vi "公式写入.vi"(7 "公式":cluster{"X^2":dbl, "X":dbl, "b":dbl}, 8 "error in (no error)":errorcluster caption="错误输入（无错误）", 9 "量程":enum16{"低量程", "高量程"}(ring), 10 "测量模式":T1(ring), 11 "测量参数":u16(ring) items=["总磷"=1, "总氮"=2, "氨氮"=3, "COD"=22]) -> (0 "error out":errorcluster caption="错误输出")   [LabVIEW 2016, in "斯坦道总氮.lvlib"]
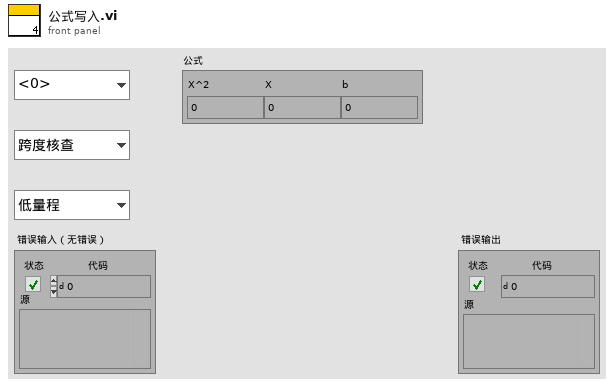
[diagram p1: front panel]
types:
  T1 = enum16{"跨度核查", "水样测量", "零点核查", "标样核查", "加标回收", "平行样测试", "空白校准", "标样校准", "空白测试"}
  T2 = typedef "SingleStepTestV3.lvlib/SingleStepTestV3.lvclass/仪器版本.ctl" = enum16{"V3.1版", "V4版", "V3版", "V4.2版"}
  T3 = cluster{"测量参数":u16, "测量模式":enum16{"跨度核查", "水样测量", "零点核查", "标样核查", "加标回收", "平行样测试", "空白校准", "标样校准", "空白测试"}, "量程":enum16{"低量程", "高量程"}}
  T4 = typedef "斯坦道总氮.lvlib/校准参数.ctl" = cluster{"公式写入时间":timestamp, "id":u8, "fid":u8, "range":u8, "拟合方法":u16, "精度":u16, "公式A":sgl, "公式B":sgl, "公式C":sgl, "R2":sgl, "校准值一":cluster{"标准值":sgl, "吸光值":sgl, "启用":bool, "数据时间":timestamp}, "校准值二":cluster{"标准值":sgl, "吸光值":sgl, "启用":bool, "数据时间":timestamp}, "校准值三":cluster{"标准值":sgl, "吸光值":sgl, "启用":bool, "数据时间":timestamp}, "校准值四":cluster{"标准值":sgl, "吸光值":sgl, "启用":bool, "数据时间":timestamp}, "校准值五":cluster{"标准值":sgl, "吸光值":sgl, "启用":bool, "数据时间":timestamp}}
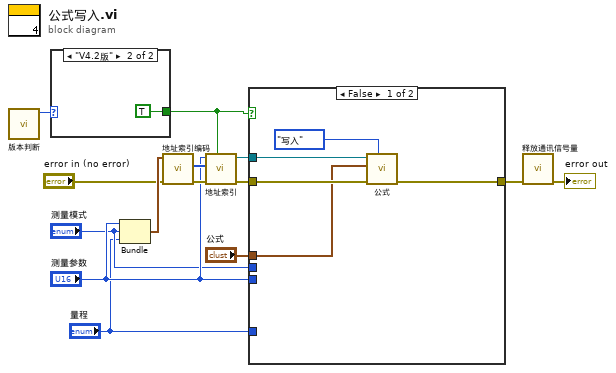
[diagram p0: block diagram]
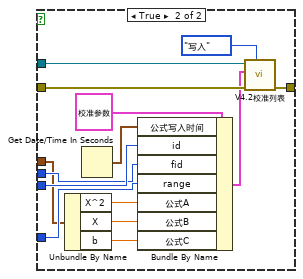
[diagram p2: hidden frame]
diagram:
  n1 = call "版本判断.vi"() -> ("仪器版本"=w9:T2)  [unwired: 11 in]
  n2 = case shown="\"V4.2版\"" w9 {
    tunnel: [_ TRUE] -> w4
    frame "V3.1版", Default {
    }
    frame "V4.2版" {
    }
  }
  n3 = Bundle("测量参数"="测量参数", "测量模式"="测量模式", "量程"="量程") -> (w8:T3)  [unwired: 1 in]
  n4 = call "地址索引编码.vi"("error in (no error)"="error in (no error)", "参数簇"=w8) -> ("error out"=w5:errorcluster, "数组"=w7:u16[])  [unwired: 8 in]
  n5 = call "地址索引.vi"("4.2写公式？"=w4, "error in (no error)"=w5, "values"=w7, "测量参数"="测量参数") -> ("error out"=w13:errorcluster, "MB session out"=w14:refnum<class "MB_Master.lvclass">)  [unwired: 6 in]
  n6 = case shown="False" w4 {
    tunnel: w14 -> [w20 w31]
    tunnel: w13 -> [w19 w34]
    tunnel: [w17 w33] -> w12
    tunnel: "公式" -> [w16 w24]
    tunnel: "测量参数" -> [_ w27]
    tunnel: "测量模式" -> [_ w26]
    tunnel: "量程" -> [_ w25]
    frame False {
      n7 = call "公式.vi"("功能"=enum16{"读取", "写入"}."写入", "error in (no error)"=w19, "公式写入"=w16, "MB session in"=w20) -> ("error out"=w17:errorcluster)  [unwired: 5 in, 2 out]
    }
    frame True {
      n8 = Unbundle By Name(w24) -> ("X^2"=w23:dbl, "X"=w22:dbl, "b"=w21:dbl)
      n9 = Get Date/Time In Seconds() -> (seconds since 1Jan1904=w28:timestamp)
      n10 = Bundle By Name(cluster=T4 {"公式写入时间"=timestamp(0 s since 1904-01-01), "id"=0, "fid"=0, "range"=0, "拟合方法"=0, "精度"=0, "公式A"=0.0, "公式B"=0.0, "公式C"=0.0, "R2"=0.0, "校准值一"={"标准值"=0.0, "吸光值"=0.0, "启用"=FALSE, "数据时间"=timestamp(0 s since 1904-01-01)}, "校准值二"={"标准值"=0.0, "吸光值"=0.0, "启用"=FALSE, "数据时间"=timestamp(0 s since 1904-01-01)}, "校准值三"={"标准值"=0.0, "吸光值"=0.0, "启用"=FALSE, "数据时间"=timestamp(0 s since 1904-01-01)}, "校准值四"={"标准值"=0.0, "吸光值"=0.0, "启用"=FALSE, "数据时间"=timestamp(0 s since 1904-01-01)}, "校准值五"={"标准值"=0.0, "吸光值"=0.0, "启用"=FALSE, "数据时间"=timestamp(0 s since 1904-01-01)}} ("校准参数 in"), "公式写入时间"=w28, "id"=w27, "fid"=w26, "range"=w25, "公式A"=w23, "公式B"=w22, "公式C"=w21) -> (w29:T4)
      n11 = call "V4.2校准列表.vi"("功能"=enum16{"读取", "写入"}."写入", "error in (no error)"=w34, "校准参数 in"=w29, "MB session in"=w31) -> ("error out"=w33:errorcluster)  [unwired: 5 in, 2 out]
    }
  }
  n12 = call "释放通讯信号量.vi"("error in (no error)"=w12) -> ("error out"=→"error out":errorcluster)  [unwired: 10 in]
